vi "Plot Load maker V2 - scalewrite.vi"(7 "Meta LUT":refnum<data-value>, 8 "error in (no error)":errorcluster, 10 "Axis config":T1={"Name Label.Text"="", "Style"=0, "Tick Colors:Minor Tick Color"=0, "Tick Colors:Tick Color"=0, "Marker Colors:Text Color"=0, "Grid Colors:Major Color"=0, "Grid Colors:Minor Color"=0, "Mapping Mode"=0, "Flipped"=FALSE, "Name Label.Visible"=FALSE, "Name Label.Text Colors:Text Color"=0, "Scale Fit"=0, "Range:Maximum"=0.0, "Range:Minimum"=0.0, "Offset and Multiplier:Multiplier"=0.0, "Offset and Multiplier:Offset"=0.0, "Name Label.Font:Size"=0, "Marker.Font:Size"=0, "Uniform Marker Spacing?"=TRUE, "Format String"=""}, 11 "Scale reference":refnum<vi>) -> (0 "error out":errorcluster, 3 "Scale reference":refnum<vi>)   [LabVIEW 2021, in "RocketPlot.lvlib"]
uses:
  RocketPlot.lvlib
  TypeDefs/Plot scale axis properties.ctl
  Plot scale refnum to LUT name.vi
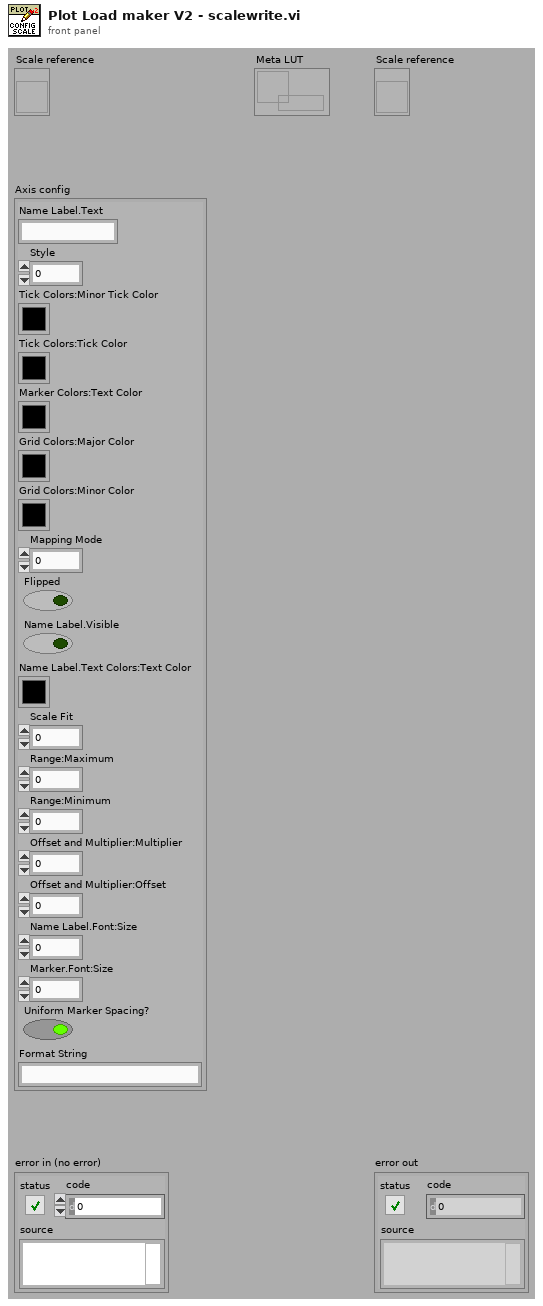
[diagram p1: front panel]
types:
  T1 = typedef "RocketPlot.lvlib/Plot scale axis properties.ctl" = cluster{"Name Label.Text":string, "Style":u8, "Tick Colors:Minor Tick Color":u32, "Tick Colors:Tick Color":u32, "Marker Colors:Text Color":u32, "Grid Colors:Major Color":u32, "Grid Colors:Minor Color":u32, "Mapping Mode":u8, "Flipped":bool, "Name Label.Visible":bool, "Name Label.Text Colors:Text Color":u32, "Scale Fit":u8, "Range:Maximum":dbl, "Range:Minimum":dbl, "Offset and Multiplier:Multiplier":dbl, "Offset and Multiplier:Offset":dbl, "Name Label.Font:Size":u32, "Marker.Font:Size":u32, "Uniform Marker Spacing?":bool, "Format String":string}
  T2 = typedef "RocketPlot.lvlib/Plot scale meta JSON.ctl" = cluster{"Type":T3, "Grid Colors:Major Color":u32, "Grid Colors:Minor Color":u32, "Style":u8, "Tick Colors:Tick Color":u32, "Tick Colors:Minor Tick Color":u32, "Format String":string, "State":T4, "AxisFocus":refnum<vi>}
  T3 = typedef "RocketPlot.lvlib/Plot axis.ctl" = enum16{"x axis", "left axis", "right axis"}
  T4 = typedef "RocketPlot.lvlib/Plot scale meta state.ctl" = cluster{"Visible":bool, "Focus":bool, "Multi-Y":bool}
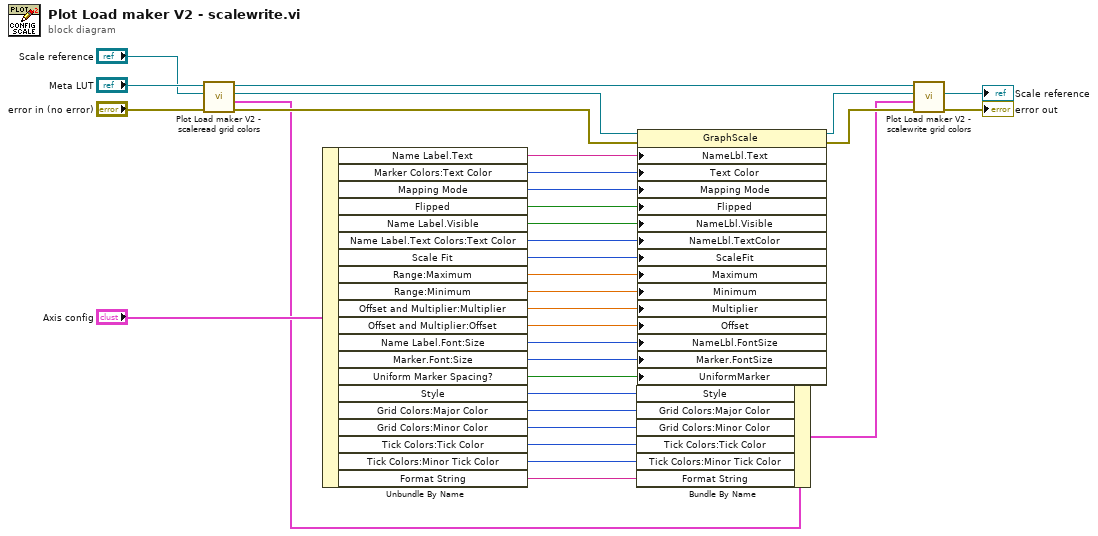
[diagram p0: block diagram]
diagram:
  n1 = call "Plot Load maker V2 - scaleread grid colors.vi"("error in (no error)"="error in (no error)", "Scale reference"="Scale reference", "Meta LUT"="Meta LUT") -> ("error out"=w2:errorcluster, "Scale LUT meta"=w1:T2, "Scale reference"=w4:refnum<vi>, "Meta LUT"=w5:refnum<data-value>)  [unwired: 5 in]
  n2 = Unbundle By Name("Axis config") -> ("Name Label.Text"=w32:string, "Marker Colors:Text Color"=w31:u32, "Mapping Mode"=w30:u8, "Flipped"=w29:bool, "Name Label.Visible"=w28:bool, "Name Label.Text Colors:Text Color"=w27:u32, "Scale Fit"=w26:u8, "Range:Maximum"=w25:dbl, "Range:Minimum"=w24:dbl, "Offset and Multiplier:Multiplier"=w23:dbl, "Offset and Multiplier:Offset"=w22:dbl, "Name Label.Font:Size"=w21:u32, "Marker.Font:Size"=w20:u32, "Uniform Marker Spacing?"=w19:bool, "Style"=w12:u8, "Grid Colors:Major Color"=w18:u32, "Grid Colors:Minor Color"=w17:u32, "Tick Colors:Tick Color"=w10:u32, "Tick Colors:Minor Tick Color"=w9:u32, "Format String"=w8:string)
  n3 = Bundle By Name(cluster=w1, "Style"=w12, "Grid Colors:Major Color"=w18, "Grid Colors:Minor Color"=w17, "Tick Colors:Tick Color"=w10, "Tick Colors:Minor Tick Color"=w9, "Format String"=w8) -> (w14:T2)
  n4 = property class="GraphScale"(reference=w4, error in=w2, "NameLbl.Text"=w32, "Text Color"=w31, "Mapping Mode"=w30, "Flipped"=w29, "NameLbl.Visible"=w28, "NameLbl.TextColor"=w27, "ScaleFit"=w26, "Maximum"=w25, "Minimum"=w24, "Multiplier"=w23, "Offset"=w22, "NameLbl.FontSize"=w21, "Marker.FontSize"=w20, "UniformMarker"=w19) -> (reference out=w15:refnum<vi>, error out=w16:errorcluster)
  n5 = call "Plot Load maker V2 - scalewrite grid colors.vi"("error in (no error)"=w16, "Meta"=w14, "Scale reference"=w15, "Meta LUT"=w5) -> ("error out"=→"error out":errorcluster, "Scale reference"=→"Scale reference":refnum<vi>)  [unwired: 5 in, 1 out]
